vi "Fpga_v3.vi"() -> ()   [LabVIEW 2015]
uses:
  <vilib>/Platform/TimedLoop/XDataNode/timing_clust.ctl
  <vilib>/Platform/TimedLoop/XDataNode/nitl_modes.ctl
  <vilib>/Platform/TimedLoop/XDataNode/wakeup.ctl
  <vilib>/rvi/Emulation/niFpgaGetClockAttributes.vi
  <vilib>/rvi/Emulation/niFpgaSctlEmulationGetInTimedLoop.vi
  <vilib>/rvi/Emulation/niFpgaEmulationReportErrorSimple.vi
  <vilib>/rvi/eio/common/nirviEmuTemplateMethod_errors.vi
  <vilib>/rvi/Emulation/niFpgaCriticalErrorInLSC.vi
  <vilib>/rvi/interface/RandomDataEmulation/niFpgaRandomDataHandleErrors.vi
  <vilib>/eio/EIONode/EIONode.xnode
  <vilib>/Platform/TimedLoop/XDataNode/XDataNode.xnode
  <vilib>/rvi/DataTransferAndStorage/Container/XNode/niFpgaContainer.xnode
  <vilib>/rvi/interface/RandomDataEmulation/nirviRandomDataFpgaReadWriteTemplate.vi
  <vilib>/Platform/TimedLoop/XDataNode/XDNodeRunTimeDep.lvlib
panel:
  in  "stop":bool
  out "x-y 3":u32
  in  "Data write ON/OFF":bool
  out "Mod2/DIO6_B":bool
  out "Timed Out?":bool
  in  "Mod4/AO0 2":i16
  out "Mod3/AI0 2":fxp<+/-,16,5>
  out "Boolean 2":bool
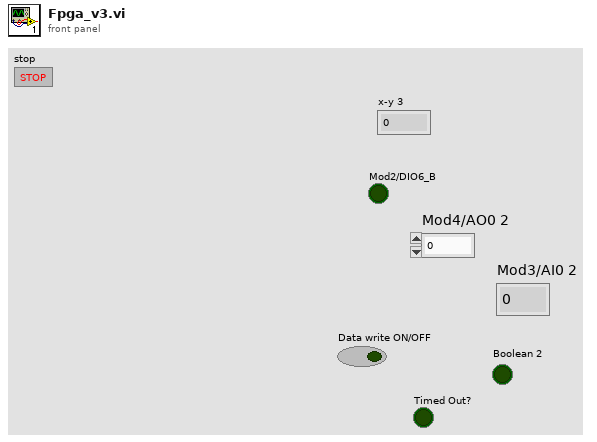
[diagram p1: front panel]
types:
  T1 = typedef "XDNodeRunTimeDep.lvlib/timing_clust.ctl" = cluster{"Expected End [f-1]":u64, "Actual End [f-1]":u64, "Finished Late? [f-1]":bool, "Expected End [i-1]":u64, "Actual End [i-1]":u64, "Finished Late? [i-1]":bool, "Expected Start [i]":u64, "Actual Start [i]":u64, "Expected Start [f]":u64, "Actual Start [f]":u64, "Source Name":string, "Structure Name":string, "Period":i64, "Deadline":i64, "Offset":i64, "Start":i64, "Priority":i32, "Timeout":i32, "Mode":T2, "Wakeup Reason":T3, "Error":errorcluster, "Source Type":string, "Secondary Source Type":string, "Global End Time":u64, "Global Start Time":u64, "Frame Duration":u64, "Iteration Duration":u64, "Assigned CPU":i32, "I/O Scan Engine Mode":u32}
  T2 = typedef "XDNodeRunTimeDep.lvlib/nitl_modes.ctl" = enum32{"No Change", "Process missed periods, maintain original phase", "Discard missed periods, maintain original phase", "Process missed periods, ignore original phase", "Discard missed periods, ignore original phase"}
  T3 = typedef "XDNodeRunTimeDep.lvlib/wakeup.ctl" = enum32{"Normal", "Aborted", "Asynchronous wakeup", "Timing source error", "Timed loop error", "Timeout"}
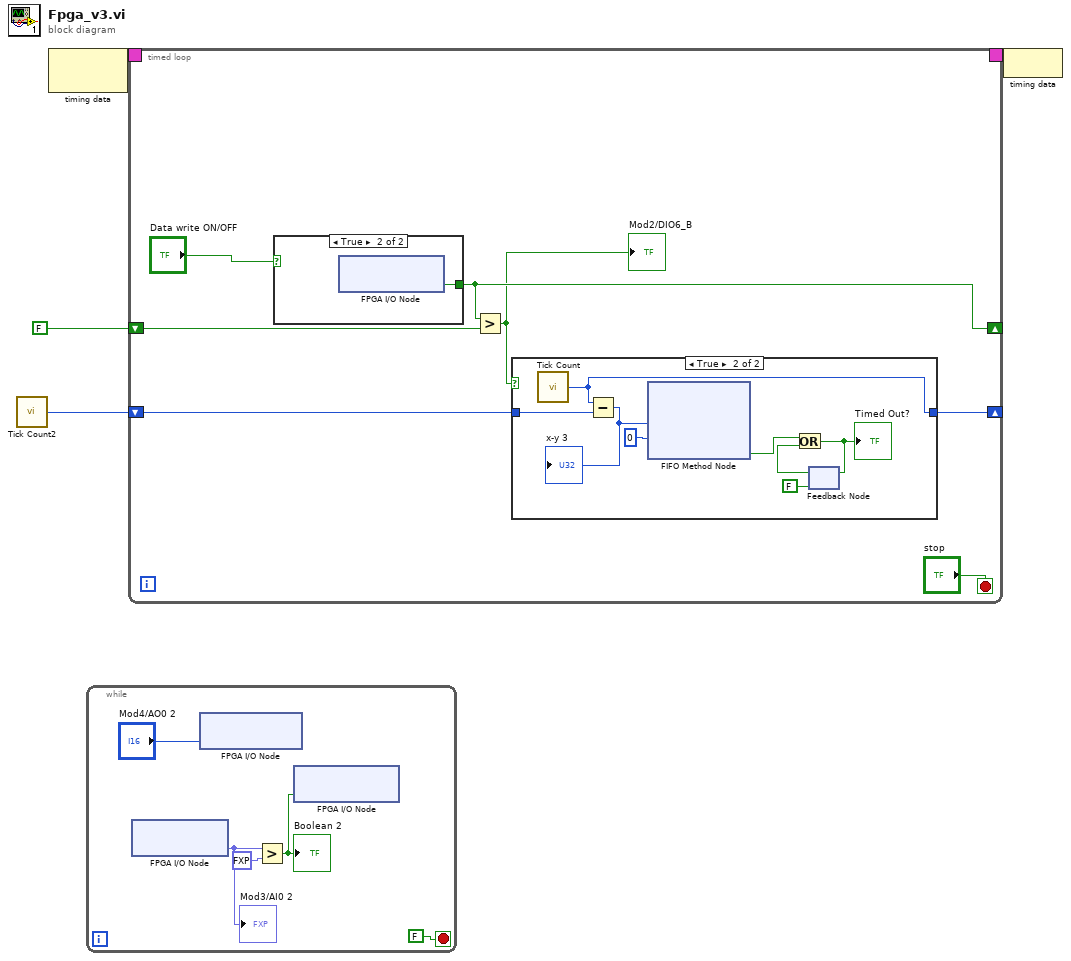
[diagram p0: block diagram]
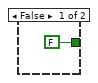
[diagram p3: hidden frame]
diagram:
  n1 = call "Tick Count2"() -> ("Tick Count(Ticks)"=w4:u32)
  n2 = node-c288() -> (w2:T1)  [unwired: 1 in]
  n3 = while {
    stop <- FALSE stop-if-true
    n4 = xnode "FPGA I/O Node"() -> ("Mod3/AI0"=w7:fxp<+/-,16,5>)  [unwired: 1 in, 1 out]
    "Mod3/AI0 2" <- w7
    n5 = xnode "FPGA I/O Node"("Mod4/AO0"="Mod4/AO0 2") -> ()  [unwired: 1 in, 1 out]
    n6 = Greater?(x=w7, y=fxp<+/-,16,5> 2.0) -> (0:w9:bool)
    "Boolean 2" <- w9
    n7 = xnode "FPGA I/O Node"("Mod2/DIO0"=w9) -> ()  [unwired: 1 in, 1 out]
  }
  n8 = timed-loop {
    shift-right: [w13] -> _
    shift-left: w4 -> [w14]
    shift-right: [w15] -> _
    shift-left: FALSE -> [w16]
    timing: w2 -> [_]
    timing-out: [_] -> w1
    stop <- "stop" stop-if-true
    n9 = case shown="True" "Data write ON/OFF" {
      tunnel: [FALSE ("Mod2/DIO6") w27] -> w15
      frame False {
      }
      frame True {
        n10 = xnode "FPGA I/O Node"() -> ("Mod2/DIO6"=w27:bool)  [unwired: 1 in, 1 out]
      }
    }
    n11 = Greater?(x=w15, y=w16) -> (0:w12:bool)
    "Mod2/DIO6_B" <- w12
    n12 = case shown="True" w12 {
      tunnel: w14 -> [w17 w20]
      tunnel: [w17 w19] -> w13
      frame False {
      }
      frame True {
        n13 = call "Tick Count"() -> ("Tick Count(Ticks)"=w19:u32)
        n14 = Subtract(x=w19, y=w20) -> (x-y=w18:u32)
        "x-y 3" <- w18
        n15 = xnode ("FIFO Method Node")("Element"=w18, "Timeout"=0) -> ("Timed Out?"=w24:bool)  [unwired: 1 in, 1 out]
        n16 = feedback #1(FALSE) -> (w23:bool)
        n17 = Or(x=w24, y=w23) -> (x .or. y?=w21:bool)
        "Timed Out?" <- w21
        n18 = feedback-in #1(w21) -> ()
      }
    }
  }
  n19 = node-c288(w1) -> ()
